vi "func_popup.vi"() -> (2 "y_vals":dbl[](array[numeric])=[1.0, 4.0, 9.0, 16.0, 25.0, 36.0, 49.0, 64.0, 81.0, 100.0], 3 "cancelled":bool)   [LabVIEW 2017, in "tools.lvlib"]
uses:
  tools.lvlib
panel:
  in  "Cancel":bool
  in  "N":i32=10
  in  "dx":dbl=1.0 format="%#_12g"
  in  "x0":dbl=1.0 format="%#_12g"
  in  "func":string="x^2 " caption="y = f(x)"
  in  "OK Button":bool
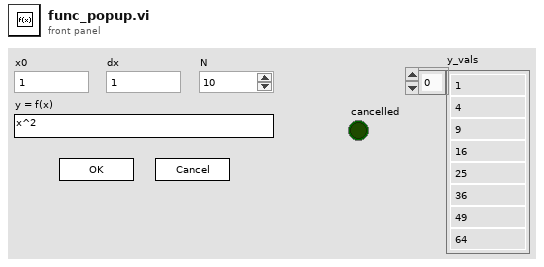
[diagram p1: front panel]
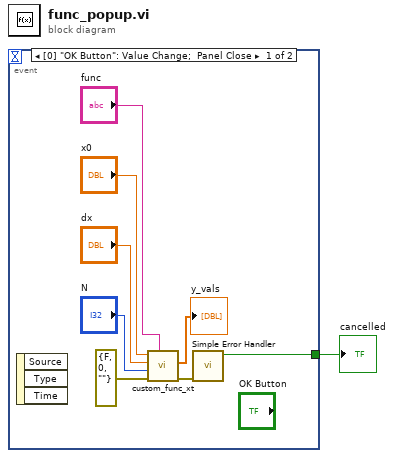
[diagram p0: block diagram]
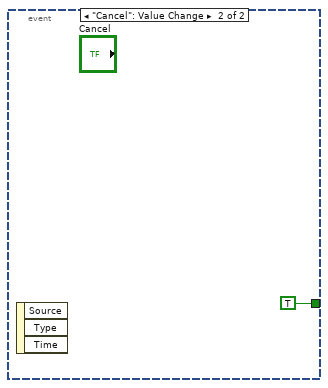
[diagram p2: hidden frame]
diagram:
  n1 = event shown="[0] \"OK Button\": Value Change;  Panel Close" {
    selector: _ -> [_ _]
    dyn-events: _ -> [_ _]
    timeout: _ -> [_ _]
    tunnel: [w2 TRUE ("Cancel")] -> w1
    event "OK Button": Value Change; Panel Close {
      n2 = event-data() -> ()  [unwired: 1 in, 3 out]
      n3 = call "custom_func_xt.vi"("func"="func", "error in (no error)"=errorcluster {"status"=FALSE, "code"=0, "source"=""}, "N"="N", "dx"="dx", "x0"="x0") -> ("error out"=w3:errorcluster, "y_vals"=→"y_vals":dbl[])  [unwired: 5 in]
      n4 = call <vilib>:"Simple Error Handler.vi"("error in (no error)"=w3) -> ("error?"=w2:bool)  [unwired: 4 in, 4 out]
    }
    event "Cancel": Value Change {
      n5 = event-data() -> ()  [unwired: 1 in, 3 out]
    }
  }
  "cancelled" <- w1
